vi "Drive Immediate.vi"(6 "Deadband Value":dbl=0.01, 7 "Description":string, 8 "Rotation":dbl, 9 "x_axis":dbl, 10 "y_axis":dbl, 11 "Operation":T1=enum."Immediate") -> (0 "Command Info Out":T2)   [LabVIEW 2017]
doc: "Often used for joystick control, this VI checks to see that the joystick axes are outside the deadband and updates the motors appropriately."
uses:
  <vilib>/Rock Robotics/WPI/Framework/Command Status Info.ctl
  <vilib>/Rock Robotics/WPI/Framework/Completion Status.ctl
  <vilib>/Rock Robotics/WPI/Framework/Completion Notifier.ctl
  Implementation/Drive Operations.ctl
  Implementation/Drive Setpoints.ctl
panel:
  in  "Command Info In":T2
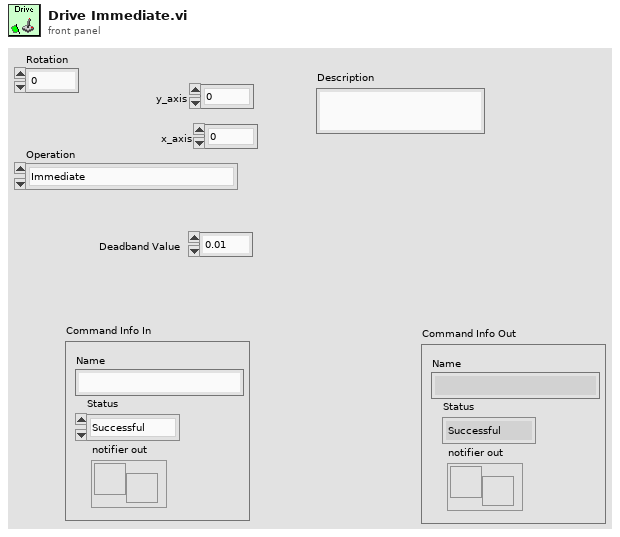
[diagram p1: front panel]
types:
  T1 = typedef "Drive Operations.ctl" = enum16{"Reserve", "Read Current", "Immediate", "Drive for Time", "Drive for Distance"}
  T2 = typedef "Command Status Info.ctl" = cluster{"Name":string, "Status":T3, "notifier out":T4}
  T3 = typedef "Completion Status.ctl" = enum16{"Successful", "Aborted", "Incomplete"}
  T4 = typedef "Completion Notifier.ctl" = refnum<notifier>
  T5 = typedef "Drive Setpoints.ctl" = cluster{"Operation":T1, "x_axis":dbl, "Rotation":dbl, "y_axis":dbl}
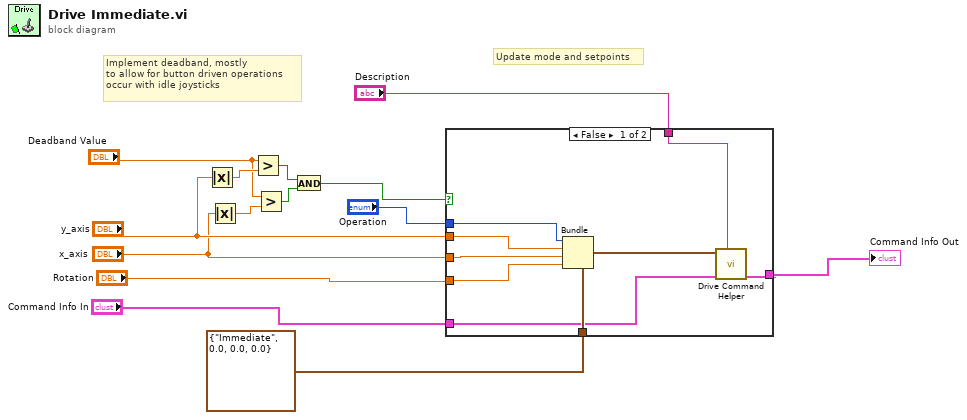
[diagram p0: block diagram]
diagram:
  # "Implement deadband, mostly\nto allow for button driven operations\noccur with idle joysticks"
  # "Update mode and setpoints"
  n1 = Absolute Value(x="y_axis") -> (abs(x)=w14:dbl)
  n2 = Absolute Value(x="x_axis") -> (abs(x)=w6:dbl)
  n3 = Greater?(x="Deadband Value", y=w14) -> (0:w8:bool)
  n4 = Greater?(x="Deadband Value", y=w6) -> (0:w4:bool)
  n5 = And(x=w8, y=w4) -> (x .and. y?=w7:bool)
  n6 = case shown="False" w7 {
    tunnel: "y_axis" -> [w23 _]
    tunnel: T5 {"Operation"=enum."Immediate", "x_axis"=0.0, "Rotation"=0.0, "y_axis"=0.0} ("SubSystem Data") -> [w22 _]
    tunnel: [w21 w24] -> w13
    tunnel: "Command Info In" -> [w20 w24]
    tunnel: "Description" -> [w18 _]
    tunnel: "x_axis" -> [w16 _]
    tunnel: "Operation" -> [w17 _]
    tunnel: "Rotation" -> [w15 _]
    frame False {
      n7 = Bundle(cluster=w22, "Operation"=w17, "x_axis"=w23, "Rotation"=w16, "y_axis"=w15) -> (w19:T5)
      n8 = call "Drive Command Helper.vi"("Description"=w18, "Command Info In"=w20, "SubSystem Data"=w19) -> ("Command Info Out"=w21:T2)  [unwired: 6 in, 2 out]
    }
    frame True {
    }
  }
  "Command Info Out" <- w13
